vi "Get IA Test Timing.vi"(8 "error in (no error)":errorcluster, 11 "IA Test Parameters in":refnum<class "IA Test Parameters.lvclass">) -> (0 "error out":errorcluster, 1 "sample rate (hz)":dbl, 2 "loop wait (ms)":dbl, 3 "IA Test Parameters out":refnum<class "IA Test Parameters.lvclass">, 4 "test time (sec)":dbl, 5 "time delay (sec)":dbl=2.0)   [LabVIEW 2020, in "IA Test Parameters.lvclass"]
uses:
  IA Test Parameters.lvclass
  IA Test Parameters.lvclass/IA Test Parameters.ctl
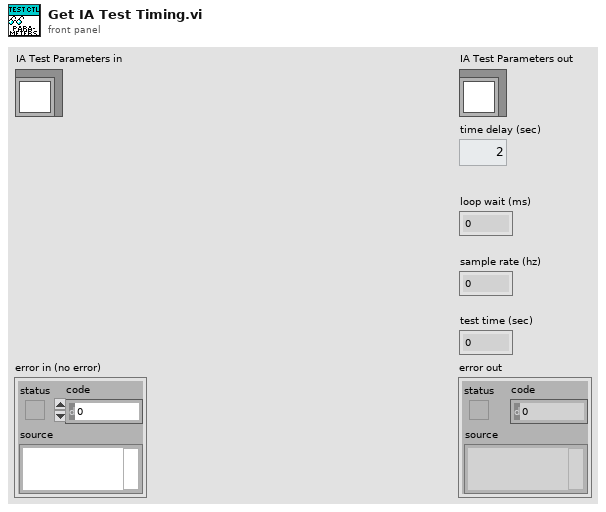
[diagram p1: front panel]
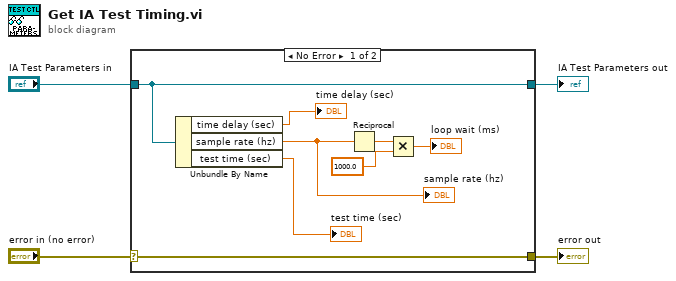
[diagram p0: block diagram]
diagram:
  n1 = case shown="No Error" "error in (no error)" {
    selector: "error in (no error)" -> [w12 w13]
    tunnel: [w12 w13] -> w3
    tunnel: [w11 w14] -> w1
    tunnel: "IA Test Parameters in" -> [w11 w14]
    frame No Error {
      n2 = Unbundle By Name(w11) -> ("time delay (sec)"=→"time delay (sec)":dbl, "sample rate (hz)"=w8:dbl, "test time (sec)"=→"test time (sec)":dbl)
      "sample rate (hz)" <- w8
      n3 = Reciprocal(x=w8) -> (1/x=w10:dbl)
      n4 = Multiply(x=w10, y=1000.0) -> (x*y=→"loop wait (ms)":dbl)
    }
    frame Error {
    }
  }
  "error out" <- w3
  "IA Test Parameters out" <- w1
